vi "Find_Optimal_Threshold.vi"(11 "0000000 4":cluster{dbl[], "Axis":dbl[]}(graph)={[0.0075, 0.0225, 0.0375, 0.0525, 0.0675, 0.08249999999999999, 0.0975, 0.11249999999999999, 0.1275, 0.14250000000000002, 0.15749999999999997, 0.1725, 0.1875, 0.2025, 0.21749999999999997, 0.23249999999999998, 0.2475, 0.2625, 0.27749999999999997, 0.2925, 0.3075, 0.3225, 0.33749999999999997, 0.3525, 0.3675, 0.3825, 0.39749999999999996, 0.4125, 0.4275, 0.4425, 0.45749999999999996, 0.4725, 0.4875, 0.5025, 0.5175000000000001, 0.5325, 0.5475, 0.5625, 0.5774999999999999, 0.5925, 0.6074999999999999, 0.6225, 0.6375, 0.6525, 0.6675, 0.6824999999999999, 0.6975, 0.7124999999999999, 0.7275, 0.7424999999999999, 0.7575000000000001, 0.7725, 0.7875, 0.8025, 0.8174999999999999, 0.8325, 0.8474999999999999, 0.8625, 0.8775, 0.8925, 0.9075, 0.9224999999999999, 0.9375, 0.9524999999999999, 0.9675, 0.9824999999999999, 0.9974999999999999, 1.0125, 1.0274999999999999, 1.0425, 1.0575, 1.0725, 1.0875, 1.1025, 1.1175, 1.1324999999999998, 1.1475, 1.1625, 1.1775, 1.1925, 1.2075, 1.2225, 1.2374999999999998, 1.2525, 1.2675, 1.2825, 1.2974999999999999, 1.3125, 1.3275, 1.3424999999999998, 1.3575, 1.3725, 1.3875, 1.4024999999999999, 1.4175, 1.4325, 1.4474999999999998, 1.4625, 1.4775, 1.4925], "Axis"=[0.0003333333333333333, 0.013000000000000001, 0.10833333333333334, 0.366, 0.6343333333333333, 0.8113333333333332, 0.9183333333333332, 0.9766666666666666, 0.9959999999999999, 0.9996666666666666, 0.9999999999999999, 0.9999999999999999, 0.9996666666666666, 0.9956666666666666, 0.9823333333333333, 0.9669999999999999, 0.9476666666666665, 0.9239999999999999, 0.8876666666666666, 0.8326666666666666, 0.7799999999999999, 0.7426666666666666, 0.7046666666666666, 0.6683333333333332, 0.6333333333333333, 0.6003333333333333, 0.5843333333333333, 0.574, 0.5599999999999999, 0.5329999999999999, 0.5119999999999999, 0.4859999999999999, 0.45766666666666656, 0.42799999999999994, 0.3963333333333333, 0.3586666666666667, 0.32400000000000007, 0.29633333333333345, 0.26866666666666683, 0.2580000000000001, 0.24966666666666681, 0.2336666666666668, 0.2223333333333335, 0.2143333333333335, 0.20733333333333348, 0.19833333333333347, 0.19000000000000017, 0.18233333333333346, 0.17466666666666675, 0.16100000000000003, 0.14066666666666672, 0.11599999999999999, 0.09699999999999998, 0.07666666666666666, 0.05599999999999994, 0.029333333333333322, 0.009666666666666601, 0.004999999999999893, 0.0009999999999998899, -1.1102230246251565e-16, -1.1102230246251565e-16, -1.1102230246251565e-16, -1.1102230246251565e-16, -1.1102230246251565e-16, -1.1102230246251565e-16, -1.1102230246251565e-16, -1.1102230246251565e-16, -1.1102230246251565e-16, -1.1102230246251565e-16, -1.1102230246251565e-16, -1.1102230246251565e-16, -1.1102230246251565e-16, -1.1102230246251565e-16, -1.1102230246251565e-16, -1.1102230246251565e-16, -1.1102230246251565e-16, -1.1102230246251565e-16, -1.1102230246251565e-16, -1.1102230246251565e-16, -1.1102230246251565e-16, -1.1102230246251565e-16, -1.1102230246251565e-16, -1.1102230246251565e-16, -1.1102230246251565e-16, -1.1102230246251565e-16, -1.1102230246251565e-16, -1.1102230246251565e-16, -1.1102230246251565e-16, -1.1102230246251565e-16, -1.1102230246251565e-16, -1.1102230246251565e-16, -1.1102230246251565e-16, -1.1102230246251565e-16, -1.1102230246251565e-16, -1.1102230246251565e-16, -1.1102230246251565e-16, -1.1102230246251565e-16, -1.1102230246251565e-16, -1.1102230246251565e-16, -1.1102230246251565e-16]}) -> (3 "Optimal Threshold":T1)   [LabVIEW 2020]
uses:
  Controls/Optimal_Threshold_Range'.ctl
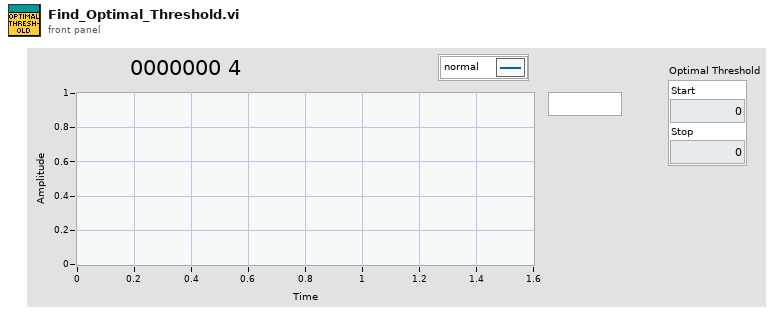
[diagram p1: front panel]
types:
  T1 = typedef "Optimal_Threshold_Range'.ctl" = cluster{"Start":dbl, "Stop":dbl}
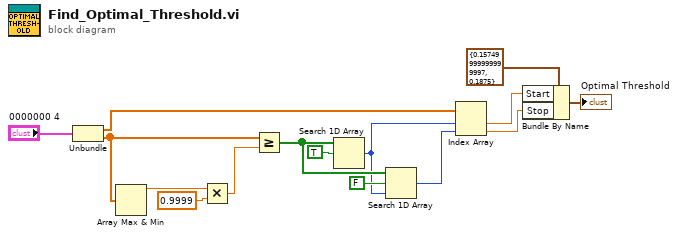
[diagram p0: block diagram]
diagram:
  n1 = Unbundle("0000000 4") -> (w11:dbl[], "Axis"=w9:dbl[])
  n2 = Array Max & Min(array=w9) -> (max value=w8:dbl)  [unwired: 3 out]
  n3 = Multiply(x=w8, y=0.9999) -> (x*y=w6:dbl)
  n4 = Greater Or Equal?(x=w9, y=w6) -> (x >= y?=w13:bool[])
  n5 = Search 1D Array(1D array=w13, element=TRUE) -> (index of element=w10:i32)  [unwired: 1 in]
  n6 = Search 1D Array(1D array=w13, element=FALSE, start index (0)=w10) -> (index of element=w5:i32)
  n7 = Index Array(array=w11, index #1=w10, index #2=w5) -> (element #1=w2:dbl, element #2=w1:dbl)
  n8 = Bundle By Name(cluster=T1 {"Start"=0.15749999999999997, "Stop"=0.1875} ("Optimal Threshold"), "Start"=w2, "Stop"=w1) -> (→"Optimal Threshold":T1)
